vi "UDP.vi"() -> ()   [LabVIEW 2014]
panel:
  in  "stop":bool
  in  "String":string
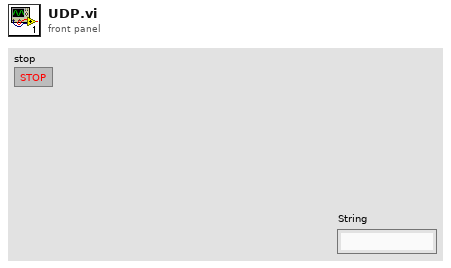
[diagram p1: front panel]
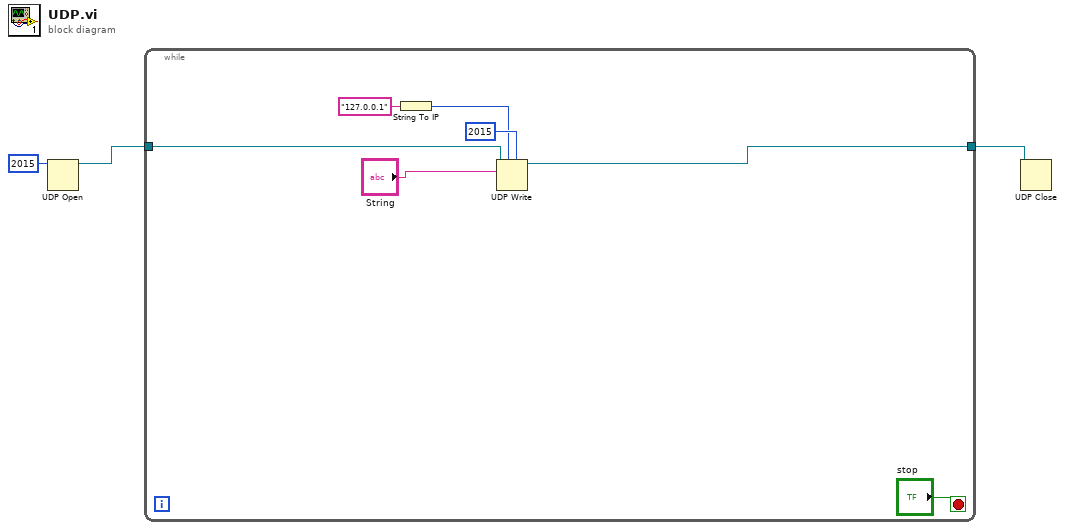
[diagram p0: block diagram]
diagram:
  n1 = UDP Open(11:u16 2015 ("port")) -> (port=w3:refnum<k16>)  [unwired: 4 in, 2 out]
  n2 = while {
    tunnel: w3 -> [w10]
    tunnel: [w9] -> w2
    stop <- "stop" stop-if-true
    n3 = String To IP(1:"127.0.0.1" ("name")) -> (0:w7:u32)
    n4 = UDP Write(address=w7, port or service name=u16 2015, connection ID=w10, data in="String") -> (3:w9:refnum<k16>)  [unwired: 2 in, 1 out]
  }
  n5 = UDP Close(connection ID=w2) -> ()  [unwired: 1 in, 2 out]
